vi "数学分析与信号处理.vi"() -> ()   [LabVIEW 2018]
panel:
  out "商 Q":dbl
  out "余数 R":dbl
  in  "停止":bool
  in  "除数 Y":dbl
  in  "被除数 X":dbl
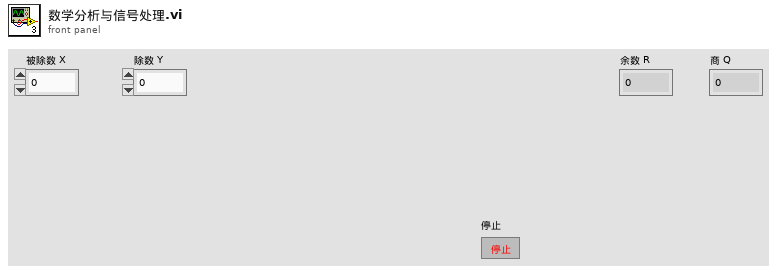
[diagram p1: front panel]
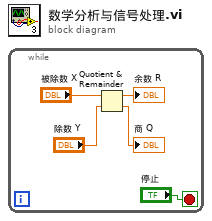
[diagram p0: block diagram]
diagram:
  n1 = while {
    stop <- "停止" stop-if-true
    n2 = Quotient & Remainder(x="被除数 X", y="除数 Y") -> (x-y*floor(x/y)=→"余数 R":dbl, floor(x/y)=→"商 Q":dbl)
  }
